vi "Begin.vi"() -> (0 "error out":errorcluster, 1 "CameraDevRef":T1)   [LabVIEW 2011]
doc: "Called before other user functions, this VI is expected to open initial I/O refnums, load in file data, and do all program initialization. Notice that the <B>error out</B> terminal is simply used for data flow. Wiring it to other structures or subVIs ensures that this VI runs first."
uses:
  <vilib>/Rock Robotics/WPI/Camera/WPI_CameraDevRef.ctl
  <vilib>/Rock Robotics/SystemInterfaces/DIO/FPGA_DIOPWMChannel.ctl
  <vilib>/Rock Robotics/WPI/Joystick/WPI_JoystickDeviceEnum.ctl
  <vilib>/Rock Robotics/SystemInterfaces/Typedef/FPGA_TypedefDigitalModule.ctl
  <vilib>/Rock Robotics/SystemInterfaces/DIO/FPGA_DIORelayChannel.ctl
  <vilib>/Rock Robotics/SystemInterfaces/AI/FPGA_AIChannel.ctl
  <vilib>/Rock Robotics/WPI/MotorControl/WPI_MotorControlOpen Victor.vi
  <vilib>/Rock Robotics/WPI/MotorControl/WPI_MotorControlOpen Jaguar.vi
  Robot Global Data.vi
panel:
  out "Global: Auton Files":string[](array[string])
  out "Global: Auton Array":dbl[][](array[numeric])
  out "Global: Current Auton File":string
  out "Global: Number of Auton Files":i64
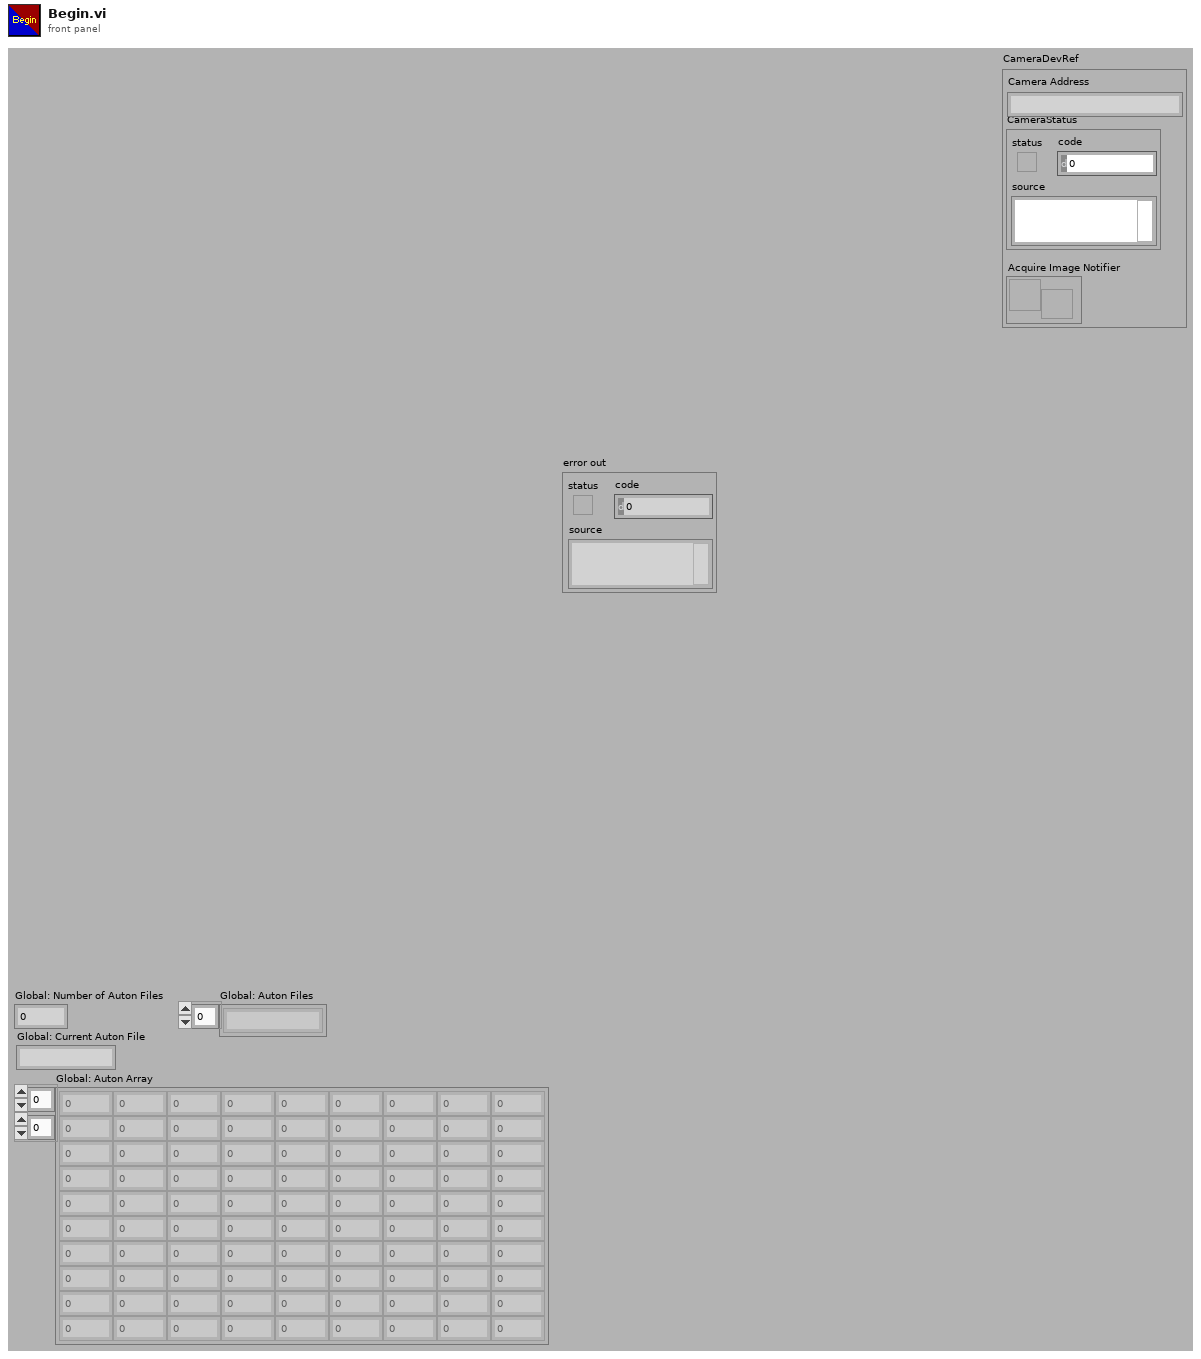
[diagram p1: front panel]
types:
  T1 = typedef "WPI_CameraDevRef.ctl" = cluster{"Camera Address":string, "CameraStatus":errorcluster, "Acquire Image Notifier":refnum<notifier>}
  T2 = typedef "FPGA_AIChannel.ctl" = enum8{"AI 1", "AI 2", "AI 3", "AI 4", "AI 5", "AI 6", "AI 7", "AI 8", "Invalid"}
  T3 = typedef "FPGA_DIORelayChannel.ctl" = enum8{"Relay 1", "Relay 2", "Relay 3", "Relay 4", "Relay 5", "Relay 6", "Relay 7", "Relay 8", "Invalid"}
  T4 = typedef "FPGA_TypedefDigitalModule.ctl" = enum16{"Digital Module 1", "Digital Module 2"}
  T5 = typedef "WPI_JoystickDeviceEnum.ctl" = enum16{"USB 1", "USB 2", "USB 3", "USB 4", "Kinect 1", "Kinect 2"}
  T6 = typedef "FPGA_DIOPWMChannel.ctl" = enum8{"PWM 1", "PWM 2", "PWM 3", "PWM 4", "PWM 5", "PWM 6", "PWM 7", "PWM 8", "PWM 9", "PWM 10", "Invalid"}
  T7 = typedef "WPI_CameraImageSize.ctl" = enum16{"640x480", "320x240", "160x120"}
  T8 = cluster{"fps":i32, "compression":i32, "Image Size":T7}
  T9 = typedef "WPI_CameraWhite Balance Values.ctl" = enum16{"Auto", "Fixed indoor", "Fixed outdoor 1", "Fixed outdoor 2", "Fixed fluorescent 1", "Fixed fluorescent 2", "Hold current"}
  T10 = typedef "WPI_ServoDeviceRef.ctl" = cluster{"DeviceStatus":errorcluster, "Digital Module":T4, "PWM Channel":T6, "DeadBand":T11}
  T11 = typedef "WPI_PWMDeadband.ctl" = cluster{"Name":string, "maxPositivePwm":i32, "minPositivePwm":i32, "centerPwm":i32, "maxNegativePwm":i32, "minNegativePwm":i32, "angularRange":u16}
  T12 = typedef "WPI_MotorControlDeviceRef.ctl" = cluster{"DeviceStatus":errorcluster, "Type":enum16{"PWM", "CAN"}, "PWM":cluster{"Digital Module":T4, "PWM Channel":T6, "DeadBand":T11}, "CAN":cluster{"Device Number":u8, "Control Mode":T13, "Semaphore":T14, "Max Vout":dbl}, "Invert":bool, "TransformRef":T15, "InvTransformRef":T15}
  T13 = typedef "WPI_CANJaguar_ControlMode.ctl" = enum8{"Percent VBus", "Current", "Speed", "Position", "Voltage"}
  T14 = typedef "Semaphore RefNum" = refnum<k1>
  T15 = typedef "WPI_PWMTransform_ConPane.ctl" = refnum<vi>
  T16 = typedef "WPI_CameraExposure Values.ctl" = enum16{"Auto", "Flicker-free 50 Hz", "Flicker-free 60 Hz", "Hold current"}
  T17 = typedef "WPI_RelayDevRef.ctl" = cluster{"DevStatus":errorcluster, "Relay Channel":T3, "Digital Module":T4, "Relay Direction":T18}
  T18 = typedef "WPI_RelayDirection.ctl" = enum16{"Both directions", "Forward only", "Reverse only"}
  T19 = typedef "WPI_JoystickDevRef.ctl" = cluster{"Device":T5}
  T20 = typedef "WPI_AnalogChannelDevRef.ctl" = cluster{"DevStatus":errorcluster, "Analog Module":T21, "Analog Channel":T2}
  T21 = typedef "FPGA_TypedefAnalogModule.ctl" = enum16{"Analog Module 1", "Analog Module 2"}
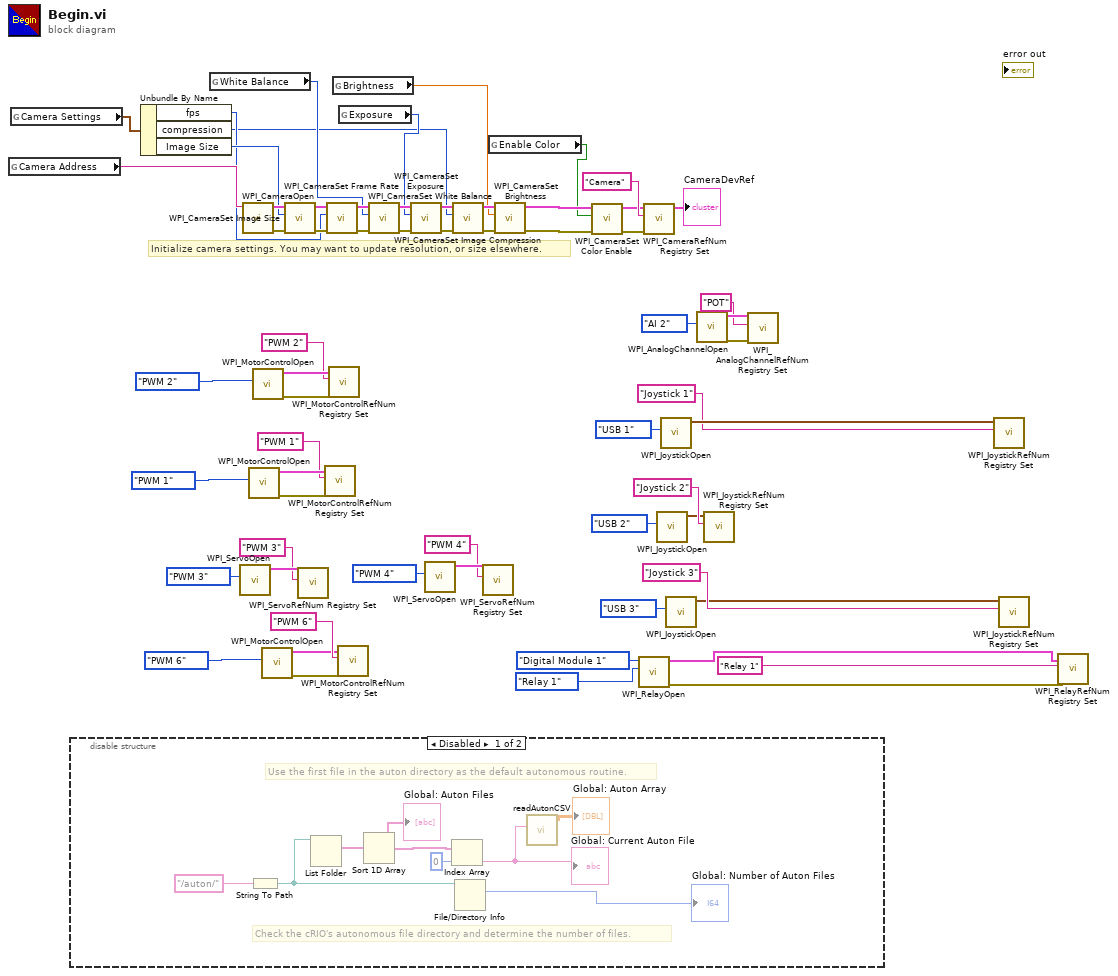
[diagram p0: block diagram]
diagram:
  # "Initialize camera settings. You may want to update resolution, or size elsewhere."
  n1 = global read "Robot Global Data.vi" "Camera Address"() -> (w50:string)
  n2 = global read "Robot Global Data.vi" "Camera Settings"() -> (w17:T8)
  n3 = disable-structure shown="Disabled" {
    frame Disabled {
      # "Check the cRIO's autonomous file directory and determine the number of files."
      # "Use the first file in the auton directory as the default autonomous routine."
      n4 = String To Path(string="/auton/") -> (path=w70:path)
      n5 = List Folder(path=w70) -> (filenames=w69:string[])  [unwired: 1 in, 5 out]
      n6 = Sort 1D Array(array=w69) -> (sorted array=w67:string[])
      "Global: Auton Files" <- w67
      n7 = Index Array(array=w67, index=0) -> (element=w65:string)
      "Global: Current Auton File" <- w65
      n8 = File/Directory Info(path=w70) -> (size=→"Global: Number of Auton Files":i64)  [unwired: 1 in, 6 out]
      n9 = call "readAutonCSV.vi"("AutonFile"=w65) -> ("AutonArray"=→"Global: Auton Array":dbl[][])  [unwired: 7 in]
    }
    frame Enabled {
    }
  }
  n10 = Unbundle By Name(w17) -> ("fps"=w15:i32, "compression"=w12:i32, "Image Size"=w16:T7)
  n11 = global read "Robot Global Data.vi" "White Balance"() -> (w14:T9)
  n12 = call <vilib>:"WPI_ServoOpen.vi"("PWM Channel"=FPGA_DIOPWMChannel."PWM 3") -> ("ServoDeviceRef"=w36:T10)  [unwired: 9 in, 1 out]
  n13 = call <vilib>:"WPI_CameraOpen.vi"("Camera Address"=w50) -> ("error out"=w56:errorcluster, "CameraDevRef"=w57:T1)  [unwired: 1 in, 8 out]
  n14 = call-poly <vilib>:"WPI_MotorControlOpen.vi"("PWM Channel"=FPGA_DIOPWMChannel."PWM 1") -> ("error out"=w42:errorcluster, "MotorControlDeviceRef"=w45:T12)  [unwired: 9 in]
  n15 = call-poly <vilib>:"WPI_MotorControlOpen.vi"("PWM Channel"=FPGA_DIOPWMChannel."PWM 2") -> ("error out"=w43:errorcluster, "MotorControlDeviceRef"=w48:T12)  [unwired: 9 in]
  n16 = call-poly <vilib>:"WPI_MotorControlOpen.vi"("PWM Channel"=FPGA_DIOPWMChannel."PWM 6") -> ("error out"=w31:errorcluster, "MotorControlDeviceRef"=w29:T12)  [unwired: 9 in]
  n17 = call <vilib>:"WPI_CameraSet Image Size.vi"("error in (no error)"=w56, "Image Size"=w16, "CameraDevRef"=w57) -> ("error out"=w55:errorcluster, "CameraDevRef Out"=w58:T1)  [unwired: 7 out]
  n18 = call <vilib>:"WPI_ServoRefNum Registry Set.vi"("refnum name"="PWM 3", "ServoDeviceRef"=w36) -> ()  [unwired: 8 in, 2 out]
  n19 = call <vilib>:"WPI_MotorControlRefNum Registry Set.vi"("error in (no error)"=w42, "refnum name"="PWM 1", "MotorControlDevRef"=w45) -> ()  [unwired: 7 in, 2 out]
  n20 = call <vilib>:"WPI_CameraSet Frame Rate.vi"("error in (no error)"=w55, "Frame Rate (fps)"=w15, "CameraDevRef"=w58) -> ("error out"=w54:errorcluster, "CameraDevRef Out"=w60:T1)  [unwired: 7 out]
  n21 = call <vilib>:"WPI_MotorControlRefNum Registry Set.vi"("error in (no error)"=w43, "refnum name"="PWM 2", "MotorControlDevRef"=w48) -> ()  [unwired: 7 in, 2 out]
  n22 = global read "Robot Global Data.vi" "Brightness"() -> (w11:dbl)
  n23 = call <vilib>:"WPI_MotorControlRefNum Registry Set.vi"("error in (no error)"=w31, "refnum name"="PWM 6", "MotorControlDevRef"=w29) -> ()  [unwired: 7 in, 2 out]
  n24 = global read "Robot Global Data.vi" "Exposure"() -> (w13:T16)
  n25 = call <vilib>:"WPI_CameraSet White Balance.vi"("error in (no error)"=w54, "White Balance"=w14, "CameraDevRef"=w60) -> ("error out"=w53:errorcluster, "CameraDevRef Out"=w59:T1)  [unwired: 7 out]
  n26 = call <vilib>:"WPI_CameraSet Exposure.vi"("error in (no error)"=w53, "Exposure"=w13, "CameraDevRef"=w59) -> ("error out"=w52:errorcluster, "CameraDevRef Out"=w62:T1)  [unwired: 7 out]
  n27 = call <vilib>:"WPI_ServoOpen.vi"("PWM Channel"=FPGA_DIOPWMChannel."PWM 4") -> ("ServoDeviceRef"=w34:T10)  [unwired: 9 in, 1 out]
  n28 = call <vilib>:"WPI_CameraSet Image Compression.vi"("error in (no error)"=w52, "Compression"=w12, "CameraDevRef"=w62) -> ("error out"=w51:errorcluster, "CameraDevRef Out"=w61:T1)  [unwired: 7 out]
  n29 = call <vilib>:"WPI_ServoRefNum Registry Set.vi"("refnum name"="PWM 4", "ServoDeviceRef"=w34) -> ()  [unwired: 8 in, 2 out]
  n30 = global read "Robot Global Data.vi" "Enable Color"() -> (w6:bool)
  n31 = call <vilib>:"WPI_CameraSet Brightness.vi"("error in (no error)"=w51, "Brightness"=w11, "CameraDevRef"=w61) -> ("error out"=w9:errorcluster, "CameraDevRef Out"=w10:T1)  [unwired: 7 out]
  n32 = call <vilib>:"WPI_CameraSet Color Enable.vi"("error in (no error)"=w9, "Color Enabled"=w6, "CameraDevRef"=w10) -> ("error out"=w7:errorcluster, "CameraDevRef Out"=w8:T1)  [unwired: 7 in]
  n33 = call <vilib>:"WPI_RelayOpen.vi"("Relay Channel"=FPGA_DIORelayChannel."Relay 1", "Digital Module (Module 1)"=FPGA_TypedefDigitalModule."Digital Module 1") -> ("error out"=w20:errorcluster, "RelayDevRef"=w21:T17)  [unwired: 8 in]
  n34 = call <vilib>:"WPI_CameraRefNum Registry Set.vi"("error in (no error)"=w7, "refnum name"="Camera", "CameraDevRef"=w8) -> ("CameraDevRef"=→"CameraDevRef":T1)  [unwired: 8 out]
  n35 = call <vilib>:"WPI_JoystickOpen.vi"("JoystickDevice"=WPI_JoystickDeviceEnum."USB 2") -> ("JoystickDevRef"=w38:T19)  [unwired: 10 in]
  n36 = call <vilib>:"WPI_JoystickOpen.vi"("JoystickDevice"=WPI_JoystickDeviceEnum."USB 1") -> ("JoystickDevRef"=w41:T19)  [unwired: 10 in]
  n37 = call <vilib>:"WPI_JoystickOpen.vi"("JoystickDevice"=WPI_JoystickDeviceEnum."USB 3") -> ("JoystickDevRef"=w26:T19)  [unwired: 10 in]
  n38 = call <vilib>:"WPI_AnalogChannelOpen.vi"("Analog Channel"=FPGA_AIChannel."AI 2") -> ("error out"=w3:errorcluster, "AIDeviceRef"=w4:T20)  [unwired: 9 in]
  n39 = call <vilib>:"WPI_JoystickRefNum Registry Set.vi"("refnum name"="Joystick 2", "JoystickDevRef"=w38) -> ()  [unwired: 8 in, 2 out]
  n40 = call <vilib>:"WPI_AnalogChannelRefNum Registry Set.vi"("error in (no error)"=w3, "refnum name"="POT", "AIDeviceRef"=w4) -> ()  [unwired: 7 in, 2 out]
  n41 = call <vilib>:"WPI_JoystickRefNum Registry Set.vi"("refnum name"="Joystick 1", "JoystickDevRef"=w41) -> ()  [unwired: 8 in, 2 out]
  n42 = call <vilib>:"WPI_JoystickRefNum Registry Set.vi"("refnum name"="Joystick 3", "JoystickDevRef"=w26) -> ()  [unwired: 8 in, 2 out]
  n43 = call <vilib>:"WPI_RelayRefNum Registry Set.vi"("error in (no error)"=w20, "refnum name"="Relay 1", "RelayDevRef"=w21) -> ()  [unwired: 7 in, 2 out]
